vi "OPCReadSQLExec.vi"() -> ()   [LabVIEW 2021]
panel:
  in  "tag":dbl
  out "Query":string caption="Result"
  out "OPC Read":dbl
  in  "stop":bool
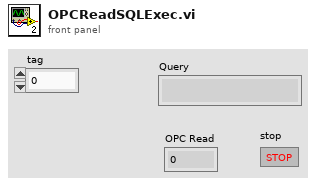
[diagram p1: front panel]
types:
  T1 = enum16{"Read", "Write", "ReadWrite", "BufferedRead", "BufferedReadWrite"}
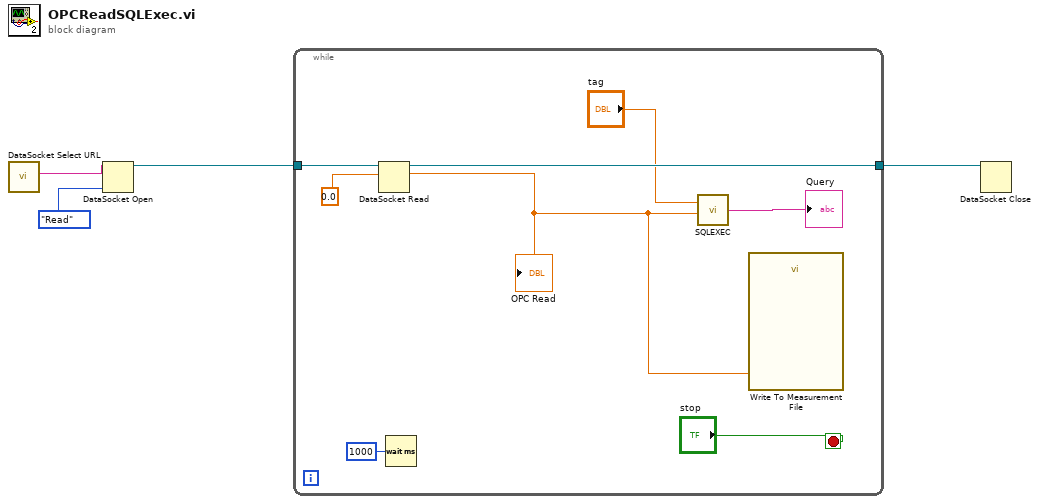
[diagram p0: block diagram]
diagram:
  n1 = call <vilib>:"DataSocket Select URL.vi"() -> ("URL"=w4:string)  [unwired: 9 in, 2 out]
  n2 = DataSocket Open(10:T1."Read" ("mode"), 11:w4) -> (3:w2:refnum<k13>)  [unwired: 2 in, 1 out]
  n3 = while {
    tunnel: w2 -> [w12]
    tunnel: [w9] -> w1
    stop <- "stop" stop-if-true
    n4 = DataSocket Read(10:0.0, 11:w12) -> (2:w5:dbl, 3:w9:refnum<k13>)  [unwired: 3 in, 5 out]
    "OPC Read" <- w5
    n5 = Wait (ms)(milliseconds to wait=u32 1000) -> ()  [unwired: 1 out]
    n6 = call "SQLEXEC.vi"("value"=w5, "tag"="tag") -> ("Query"=→"Query":string)
    n7 = call "Write To Measurement File"("Signals"=w5) -> ()  [unwired: 16 in, 3 out]
  }
  n8 = DataSocket Close(11:w1) -> ()  [unwired: 2 in, 2 out]
